vi "DataLengthBytes.vi"(10 "Is masked?":bool=TRUE, 11 "Data":string) -> (3 "Length Bytes":string)   [LabVIEW 2016, in "WebSockets.lvlib"]
doc: "Generates the message length bytes of the WebSockets packet. A varying number of bytes is used to indicate the length of the data.\nWebSockets 1.6.0.22\nSam Sharp - MediaMongrels Ltd\nCopyright (c) 2016, MediaMongrels Ltd"
uses:
  WebSockets.lvlib
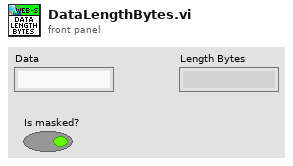
[diagram p1: front panel]
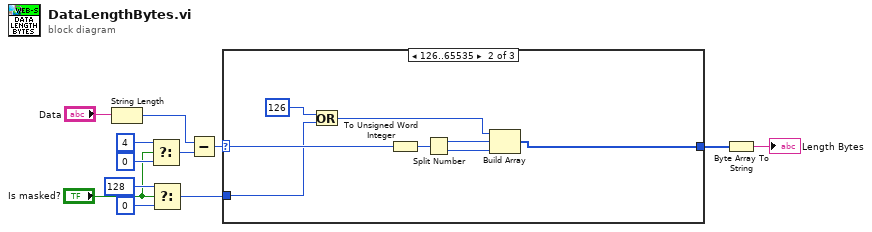
[diagram p0: block diagram]
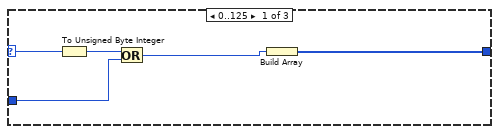
[diagram p2: hidden frame]
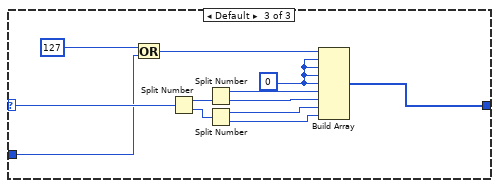
[diagram p3: hidden frame]
diagram:
  n1 = String Length(string="Data") -> (length=w6:i32)
  n2 = Select(t=4, s="Is masked?", f=0) -> (s? t:f=w1:i32)
  n3 = Select(t=u8 128, s="Is masked?", f=u8 0) -> (s? t:f=w7:u8)
  n4 = Subtract(x=w6, y=w1) -> (x-y=w5:i32)
  n5 = case shown="126..65535" w5 {
    selector: w5 -> [w14 w22 w30]
    tunnel: [w17 w21 w29] -> w11
    tunnel: w7 -> [w16 w18 w27]
    frame 0..125 {
      n6 = To Unsigned Byte Integer(number=w14) -> (unsigned 8bit integer=w15:u8)
      n7 = Or(x=w15, y=w16) -> (x .or. y?=w13:u8)
      n8 = Build Array(w13) -> (w17:u8[])
    }
    frame 126..65535 {
      n9 = Or(x=u8 126, y=w18) -> (x .or. y?=w19:u8)
      n10 = To Unsigned Word Integer(number=w22) -> (unsigned 16bit integer=w25:u16)
      n11 = Split Number(x=w25) -> (hi(x)=w24:u8, lo(x)=w23:u8)
      n12 = Build Array(w19, w24, w23) -> (w21:u8[])
    }
    frame Default {
      w31 = u8 0
      n13 = Or(x=u8 127, y=w27) -> (x .or. y?=w26:u8)
      n14 = Split Number(x=w30) -> (hi(x)=w37:u16, lo(x)=w36:u16)
      n15 = Split Number(x=w37) -> (hi(x)=w35:u8, lo(x)=w34:u8)
      n16 = Split Number(x=w36) -> (hi(x)=w33:u8, lo(x)=w32:u8)
      n17 = Build Array(w26, w31, w31, w31, w31, w35, w34, w33, w32) -> (w29:u8[])
    }
  }
  n18 = Byte Array To String(unsigned byte array=w11) -> (string=→"Length Bytes":string)
